vi "TDC_getCoincCounters.vi"(8 "Error In":errorcluster) -> (0 "Error Out":errorcluster, 3 "Coincidence Counters":i32[](array[numeric]))   [LabVIEW 2011]
uses:
  lib/tdcbase.dll
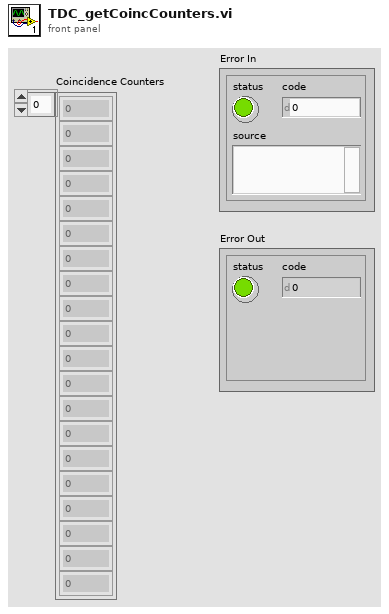
[diagram p1: front panel]
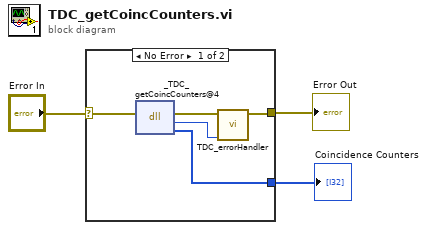
[diagram p0: block diagram]
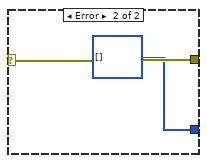
[diagram p2: hidden frame]
diagram:
  n1 = case shown="No Error" "Error In" {
    selector: "Error In" -> [w7 w10]
    tunnel: [w5 w10] -> w1
    tunnel: [w8 i32[] []] -> w2
    frame No Error {
      n2 = dll-call lib="C:/Users/hw/Documents/quTAU/userlib/lib/tdcbase.dll" fn="_TDC_getCoincCounters@4"(error in=w7) -> (error out=w6:errorcluster, "return type"=w4:i32, "data"=w8:i32[])  [unwired: 3 in, 1 out]
      n3 = call "TDC_errorHandler.vi"("quTAU Return Code"=w4, "Error In"=w6) -> ("Error Out"=w5:errorcluster)  [unwired: 9 in]
    }
    frame Error {
    }
  }
  "Error Out" <- w1
  "Coincidence Counters" <- w2
